vi "Problem_Track_Sorter-3.vi"(0 "[IN] Unsorted Tracks":dbl[][](array[numeric]), 1 "[IN] Dot matrix":i16[][](array[numeric]), 3 "error IN":errorcluster) -> (4 "Filtered Dot Stat Matrix":i16[][](array[numeric]), 5 "Sorted Tracks OUT":dbl[][](array[numeric]), 6 "Track ID OUT":u16[](array[numeric]), 7 "Start Pos OUT":i32[](array[numeric]), 8 "error OUT":errorcluster)   [LabVIEW 2013]
doc: "SubVI sorts the tracks and assigns them the same ID"
panel:
  out "ID-dot matrix OUT":u16[][](array[numeric])
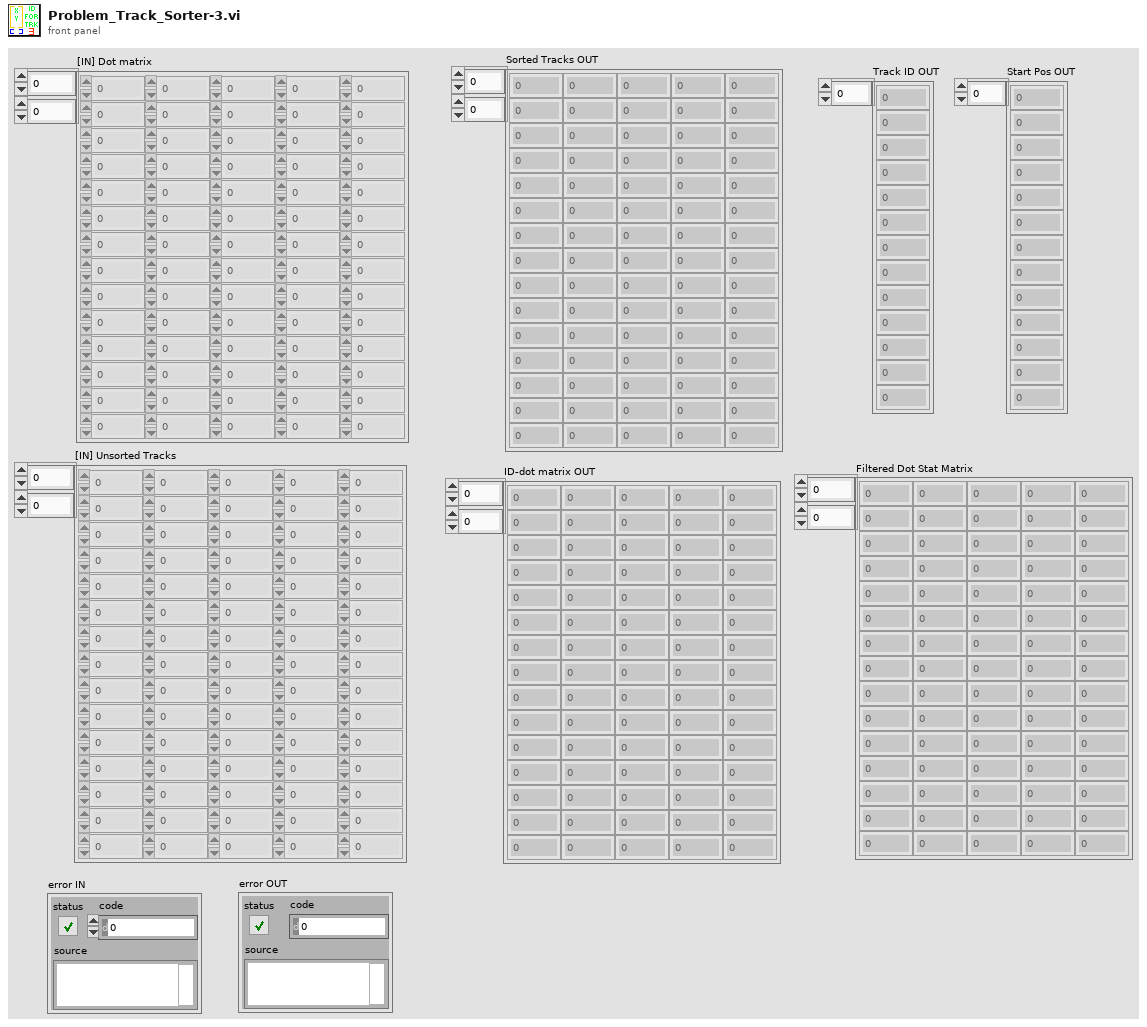
[diagram p1: front panel]
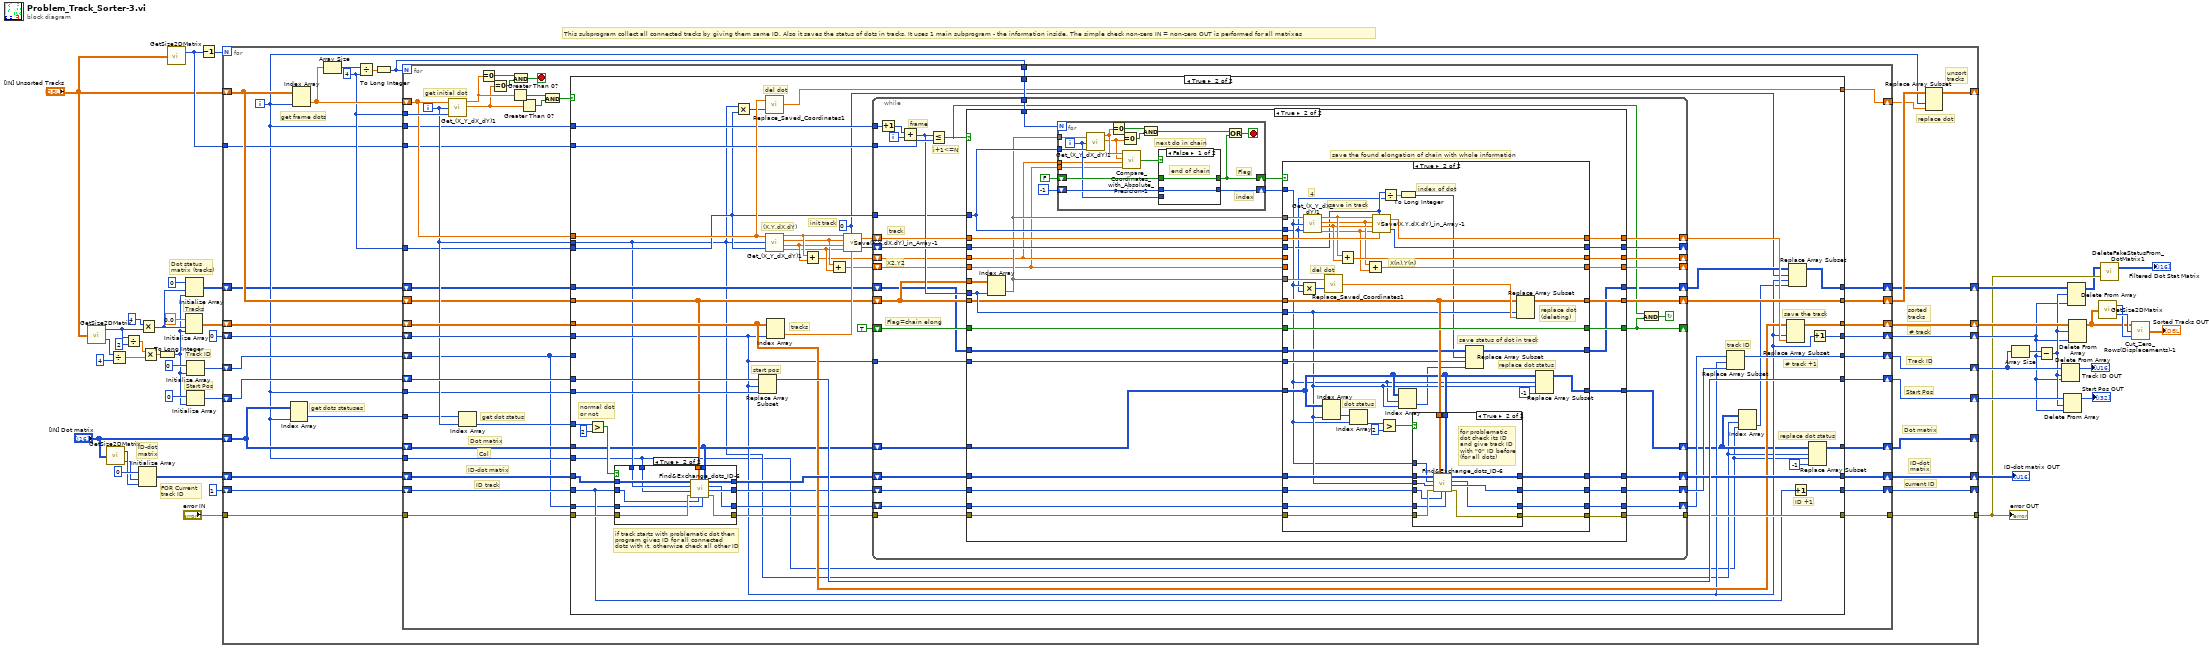
[diagram p0: block diagram]
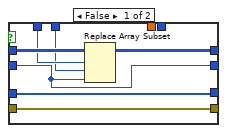
[diagram p3: hidden frame]
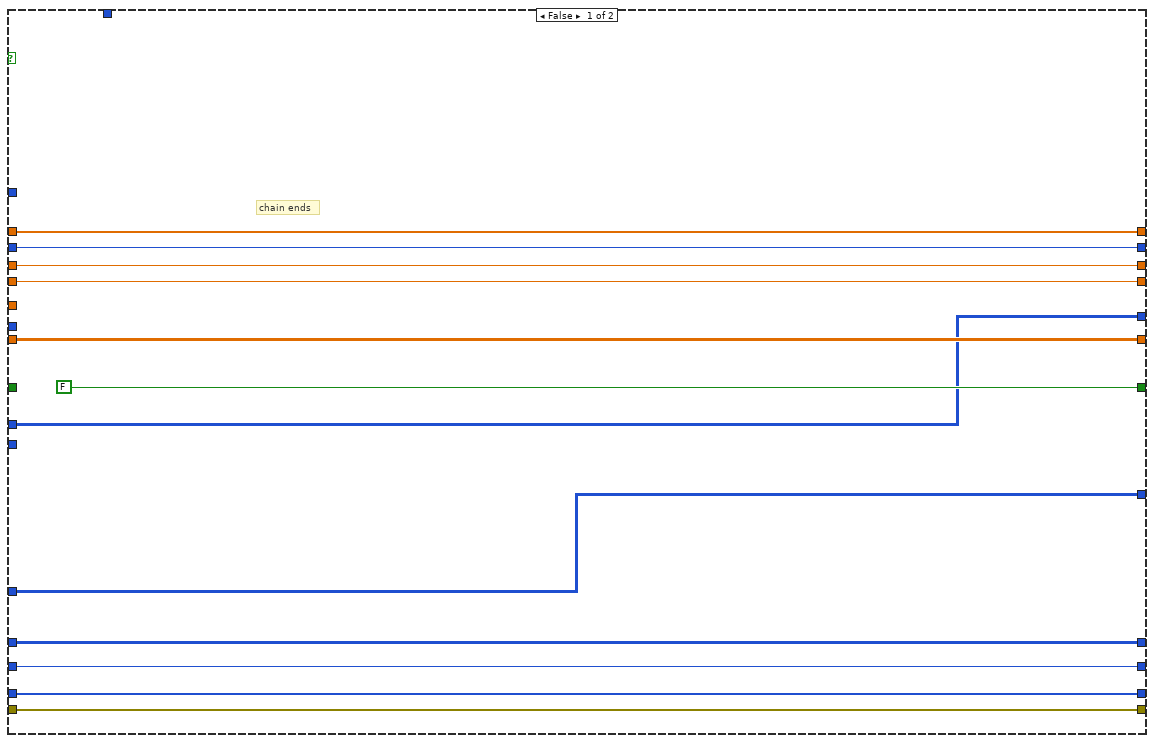
[diagram p4: hidden frame]
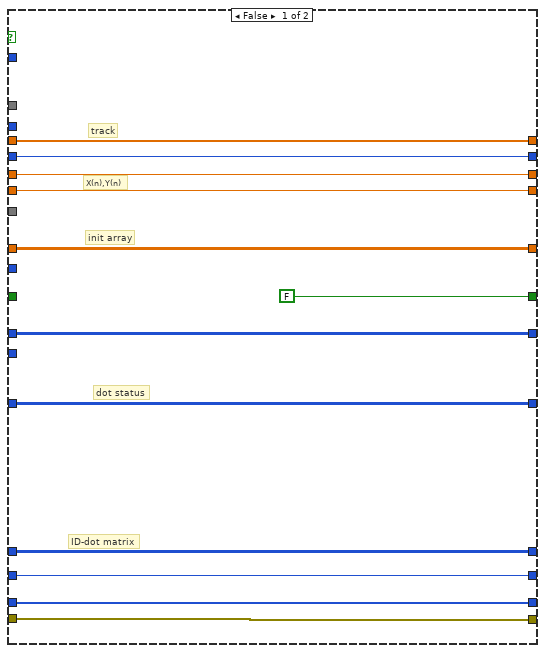
[diagram p5: hidden frame]
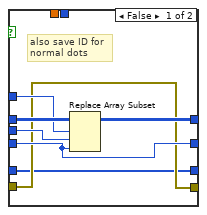
[diagram p6: hidden frame]
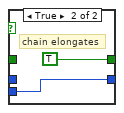
[diagram p7: hidden frame]
diagram:
  # "This subprogram collect all connected tracks by giving them same ID. Also it saves the status of dots in tracks. It uses 1 main subprogram - the information inside. The simple check non-zero IN = non-zero OUT is performed for all matrixes"
  # "Dot status\nmatrix (tracks)"
  # "FOR Current \ntrack ID"
  # "Start Pos"
  # "Track ID"
  # "Tracks"
  # "ID-dot\nmatrix"
  n1 = call "GetSize2DMatrix.vi"("Array IN (2D)"="[IN] Unsorted Tracks") -> ("# Cols"=w38:i32, "# Rows"=w40:i32)
  n2 = call "GetSize2DMatrix.vi"("Array IN (2D)"="[IN] Dot matrix") -> ("# Cols"=w44:i32, "# Rows"=w43:i32)
  n3 = Divide(x=w40, y=4) -> (x/y=w35:dbl)
  n4 = Divide(x=w38, y=2) -> (x/y=w36:dbl)
  n5 = Initialize Array(u16 0 ("element"), w43, w44) -> (w25:u16[][])
  n6 = Multiply(x=4, y=w38) -> (x*y=w10:i32)
  n7 = Multiply(x=w36, y=w35) -> (x*y=w34:dbl)
  n8 = To Long Integer(number=w34) -> (32bit integer=w9:i32)
  n9 = call "GetSize2DMatrix.vi"("Array IN (2D)"="[IN] Unsorted Tracks") -> ("# Cols"=w26:i32)  [unwired: 1 out]
  n10 = Initialize Array(0.0 ("element"), w10, w9) -> (w33:dbl[][])
  n11 = Initialize Array(i16 0, w10, w9) -> (w8:i16[][])
  n12 = Initialize Array(0 ("element"), w9) -> (w30:i32[])
  n13 = Initialize Array(u16 0 ("element"), w9) -> (w29:u16[])
  n14 = Decrement(x=w26) -> (x-1=w46:i32)
  n15 = for {
    N: w46 -> [_]
    shift-right: [w51] -> _
    shift-left: "[IN] Unsorted Tracks" -> [w65]
    shift-right: [w55] -> _
    shift-left: "[IN] Dot matrix" -> [w66]
    shift-right: [w58] -> w13
    shift-left: w33 -> [w71]
    shift-right: [w56] -> w19
    shift-left: w30 -> [w69]
    shift-right: [w57] -> w22
    shift-left: w29 -> [w70]
    shift-right: [w53] -> _
    shift-left: u16 1 -> [w72]
    shift-right: [w59] -> w5
    shift-left: 0 ("element") -> [w68]
    tunnel: w26 -> [w64]
    shift-right: [w54] -> w23
    shift-left: w25 -> [w62]
    tunnel: "error IN" -> [w61]
    tunnel: [w60] -> w4
    shift-right: [w47] -> w7
    shift-left: w8 -> [w48]
    i -> [w49]
    w67 = 4 ("y")
    # "replace dot"
    # "current ID"
    # "ID-dot\nmatrix"
    # "Dot matrix"
    # "Start Pos"
    # "Track ID"
    # "sorted \ntracks"
    # "unsort\ntracks"
    # "# track"
    # "get dots statuses"
    # "get frame dots"
    n16 = Index Array(array=w66, index (col)=w49) -> (element=w73:i16[])  [unwired: 1 in]
    n17 = Index Array(array=w65, index (col)=w49) -> (element=w74:dbl[])  [unwired: 1 in]
    n18 = Array Size(array=w74) -> (size(s)=w76:i32)
    n19 = Divide(x=w76, y=w67) -> (x/y=w75:dbl)
    n20 = To Long Integer(number=w75) -> (32bit integer=w63:i32)
    n21 = for {
      N: w63 -> [_]
      tunnel: w67 -> [w116]
      shift-right: [w84] -> w53
      shift-left: w72 -> [w92]
      shift-right: [w89] -> w58
      shift-left: w71 -> [w107]
      shift-right: [w87] -> w57
      shift-left: w70 -> [w79]
      shift-right: [w91] -> w56
      shift-left: w69 -> [w108]
      shift-right: [w88] -> w59
      shift-left: w68 -> [w106]
      tunnel: w67 -> [w101]
      shift-right: [w90] -> w52
      shift-left: w65 -> [w99]
      shift-right: [w86] -> w55
      shift-left: w66 -> [w80]
      tunnel: w49 -> [w98]
      tunnel: w49 -> [w97]
      tunnel: w64 -> [w96]
      tunnel: w63 -> [w95]
      tunnel: w49 -> [w94]
      shift-right: [w85] -> w54
      shift-left: w62 -> [w93]
      tunnel: w73 -> [w100]
      tunnel: w61 -> [w83]
      tunnel: [w82] -> w60
      shift-right: [w81] -> w50
      shift-left: w74 -> [w103]
      shift-right: [w77] -> w47
      shift-left: w48 -> [w78]
      i -> [w102]
      stop <- w113 stop-if-true
      # "Col"
      # "Dot matrix"
      # "ID-dot matrix"
      # "ID track"
      # "get dot status"
      # "get initial dot"
      n22 = call "Get_(X_Y_dX_dY)1.vi"("(X,Y,dX,dY)"=w103, "index"=w102, "multiplier"=w116) -> ("X"=w105:dbl, "Y"=w104:dbl)  [unwired: 2 out]
      n23 = Index Array(array=w100, index=w102) -> (element=w109:i16)
      n24 = Equal To 0?(x=w105) -> (x = 0?=w115:bool)
      n25 = Equal To 0?(x=w104) -> (x = 0?=w114:bool)
      n26 = Greater Than 0?(x=w105) -> (x > 0?=w112:bool)
      n27 = And(x=w115, y=w114) -> (x .and. y?=w113:bool)
      n28 = Greater Than 0?(x=w104) -> (x > 0?=w111:bool)
      n29 = And(x=w112, y=w111) -> (x .and. y?=w110:bool)
      n30 = case shown="True" w110 {
        tunnel: w109 -> [_ w182]
        tunnel: w79 -> [w123 _]
        tunnel: w108 -> [w127 w180]
        tunnel: w107 -> [w125 w151]
        tunnel: w106 -> [w124 w135]
        tunnel: w103 -> [w118 w179]
        tunnel: w102 -> [_ w131]
        tunnel: w101 -> [_ w145]
        tunnel: w80 -> [w122 w139]
        tunnel: w99 -> [w126 w144]
        tunnel: w98 -> [_ w178]
        tunnel: w97 -> [_ w177]
        tunnel: w96 -> [_ w176]
        tunnel: w95 -> [_ w175]
        tunnel: w94 -> [_ w130]
        tunnel: w93 -> [w121 w153]
        tunnel: w92 -> [w120 w143]
        tunnel: [w127 w172] -> w91
        tunnel: [w126 w174] -> w90
        tunnel: [w125 w169] -> w89
        tunnel: [w124 w168] -> w88
        tunnel: [w123 w173] -> w87
        tunnel: [w122 w138] -> w86
        tunnel: [w121 w171] -> w85
        tunnel: [w120 w170] -> w84
        tunnel: w83 -> [w119 w149]
        tunnel: [w119 w167] -> w82
        tunnel: [w118 w146] -> w81
        tunnel: w79 -> [_ w142]
        tunnel: w78 -> [w117 w137]
        tunnel: [w117 w128] -> w77
        frame False {
          # "fake dot! not counting"
        }
        frame True {
          w134 = 0
          # "if track starts with problematic dot then \nprogram gives ID for all connected\ndots with it, otherwise check all other ID"
          # "replace dot status"
          # "# track +1"
          # "ID +1"
          # "save the track"
          # "track ID"
          # "tracks"
          # "start pos"
          # "(X,Y,dX,dY)"
          # "init track"
          # "del dot"
          # "normal dot\nor not"
          n31 = Greater?(x=w182, y=i16 2) -> (0:w150:bool)
          n32 = case shown="True" w150 {
            tunnel: w143 -> [w185 w195]
            tunnel: w153 -> [w189 w199]
            tunnel: [w188 w190] -> w152
            tunnel: [w185 w192] -> w147
            tunnel: w149 -> [w184 w196]
            tunnel: [w184 w193] -> w148
            tunnel: w144 -> [_ w201]
            tunnel: w139 -> [_ w200]
            tunnel: w131 -> [w187 w198]
            tunnel: w130 -> [w186 w197]
            tunnel: [w183 w191] -> w141
            tunnel: w142 -> [w183 w194]
            frame False {
              n33 = Replace Array Subset(array=w189, new element=w185, index (row)=w187, index (col)=w186) -> (w188:u16[][])
            }
            frame True {
              n34 = call "Find&Exchange_dots_ID-6.vi"("Track ID Arr IN"=w194, "Dot matrix (stat)"=w200, "track ID IN"=w195, "(X,Y...) Tracks"=w201, "error IN"=w196, "frame (col)"=w197, "index of \ndot in frame"=w198, "ID-dot matrix"=w199) -> ("error OUT"=w193:errorcluster, "track ID OUT"=w192:u16, "Track ID Arr OUT"=w191:u16[], "ID-dot matrix OUT"=w190:u16[][])
            }
          }
          n35 = Multiply(x=w131, y=w145) -> (x*y=w165:i32)
          n36 = Replace Array Subset(array=w180, new element=w178, index=w135) -> (w172:i32[])
          n37 = call "Replace_Saved_Coordinates1.vi"("Index of staring point"=w165, "(X,Y,dX,dY) Frame IN"=w179) -> ("Replaced array"=w146:dbl[])
          n38 = call "Get_(X_Y_dX_dY)1.vi"("(X,Y,dX,dY)"=w179, "index"=w131, "multiplier"=w145) -> ("X"=w162:dbl, "Y"=w160:dbl, "dX"=w161:dbl, "dY"=w159:dbl)
          n39 = Index Array(array=w151, index (col)=w135) -> (element=w166:dbl[])  [unwired: 1 in]
          n40 = Add(x=w162, y=w161) -> (x+y=w158:dbl)
          n41 = Add(x=w160, y=w159) -> (x+y=w157:dbl)
          n42 = call "Save(X,Y,dX,dY)_in_Array-1.vi"("Array for Replacement IN"=w166, "Starting Position"=w134, "dY"=w159, "dX"=w161, "Y"=w160, "X"=w162) -> ("Finish Position"=w163:i32, "Array for Replacement OUT"=w164:dbl[])
          n43 = while {
            shift-right: [w221] -> w174
            shift-left: w144 -> [w222]
            shift-right: [w219] -> w154
            shift-left: w164 -> [w234]
            shift-right: [w218] -> _
            shift-left: w163 -> [w233]
            shift-right: [w212] -> w132
            shift-left: w139 -> [w217]
            tunnel: w177 -> [w231]
            tunnel: w176 -> [w235]
            shift-right: [w224] -> _
            shift-left: w158 -> [w228]
            shift-right: [w223] -> _
            shift-left: w157 -> [w227]
            tunnel: w175 -> [w226]
            tunnel: w145 -> [w225]
            shift-right: [w214] -> w171
            shift-left: w152 -> [w216]
            shift-right: [w210] -> _
            shift-left: TRUE -> [w220]
            shift-right: [w213] -> w155
            shift-left: w147 -> [w215]
            tunnel: w148 -> [w208]
            tunnel: [w207] -> w167
            shift-right: [w205] -> w140
            shift-left: w141 -> [w206]
            shift-right: [w202] -> w136
            shift-left: w137 -> [w204]
            tunnel: w135 -> [w203]
            i -> [w232]
            stop <- w211 continue-if-true
            # "i+1<=N"
            # "Flag=chain elong"
            # "frame"
            # "track"
            # "X2,Y2"
            n44 = Increment(x=w231) -> (x+1=w230:i32)
            n45 = Add(x=w230, y=w232) -> (x+y=w229:i32)
            n46 = Less Or Equal?(x=w229, y=w235) -> (x <= y?=w209:bool)
            n47 = case shown="True" w209 {
              tunnel: w222 -> [_ w272]
              tunnel: w234 -> [w247 w275]
              tunnel: w233 -> [w246 w274]
              tunnel: w229 -> [_ w271]
              tunnel: w228 -> [w245 w265]
              tunnel: w227 -> [w244 w264]
              tunnel: w226 -> [_ w281]
              tunnel: w225 -> [_ w276]
              tunnel: [w247 w269] -> w219
              tunnel: [w246 w268] -> w218
              tunnel: [w245 w267] -> w224
              tunnel: [w244 w266] -> w223
              tunnel: w222 -> [w243 w253]
              tunnel: [w243 w270] -> w221
              tunnel: w220 -> [_ w263]
              tunnel: [FALSE w262] -> w210
              tunnel: w217 -> [w240 w261]
              tunnel: w216 -> [w241 w260]
              tunnel: w215 -> [w239 w259]
              tunnel: [w241 w258] -> w214
              tunnel: [w239 w257] -> w213
              tunnel: [w240 w256] -> w212
              tunnel: w208 -> [w238 w255]
              tunnel: [w238 w254] -> w207
              tunnel: w206 -> [w237 w252]
              tunnel: [w237 w251] -> w205
              tunnel: w204 -> [w236 w250]
              tunnel: w203 -> [_ w249]
              tunnel: [w236 w248] -> w202
              frame False {
                # "chain ends"
              }
              frame True {
                # "save the found elongation of chain with whole information"
                n48 = Index Array(array=w272, index (col)=w271) -> (element=w273:dbl[])  [unwired: 1 in]
                n49 = for {
                  N: w281 -> [_]
                  tunnel: w273 -> [w369]
                  tunnel: w276 -> [w368]
                  tunnel: w265 -> [w356]
                  tunnel: w264 -> [w355]
                  shift-right: [w361] -> w278
                  shift-left: FALSE -> [w363]
                  shift-right: [w360] -> w277
                  shift-left: -1 -> [w362]
                  i -> [w359]
                  stop <- w364 stop-if-true
                  # "next do in chain"
                  # "index"
                  # "Flag"
                  n50 = call "Get_(X_Y_dX_dY)1.vi"("(X,Y,dX,dY)"=w369, "index"=w359, "multiplier"=w368) -> ("X"=w358:dbl, "Y"=w357:dbl)  [unwired: 2 out]
                  n51 = Equal To 0?(x=w358) -> (x = 0?=w367:bool)
                  n52 = Equal To 0?(x=w357) -> (x = 0?=w366:bool)
                  n53 = call "Compare_Coordinates_with_Absolute_Presicion-1.vi"("X 1"=w358, "Y 1"=w357, "X 2"=w356, "Y 2"=w355) -> ("[OUT] Same coordinates?"=w354:bool)  [unwired: 1 in]
                  n54 = And(x=w367, y=w366) -> (x .and. y?=w365:bool)
                  n55 = case shown="False" w354 {
                    tunnel: w363 -> [w371 _]
                    tunnel: w362 -> [w370 _]
                    tunnel: [w371 TRUE] -> w361
                    tunnel: [w370 w372] -> w360
                    tunnel: w359 -> [_ w372]
                    frame False {
                      # "end of chain"
                    }
                    frame True {
                      # "chain elongates"
                    }
                  }
                  n56 = Or(x=w365, y=w361) -> (x .or. y?=w364:bool)
                }
                n57 = case shown="True" w278 {
                  tunnel: w277 -> [_ w300]
                  tunnel: w273 -> [_ w334]
                  tunnel: w276 -> [_ w298]
                  tunnel: w275 -> [w293 w333]
                  tunnel: w274 -> [w292 w299]
                  tunnel: w273 -> [_ w331]
                  tunnel: w253 -> [w291 w307]
                  tunnel: w271 -> [_ w301]
                  tunnel: [w293 w329] -> w269
                  tunnel: [w292 w328] -> w268
                  tunnel: [w291 w311] -> w270
                  tunnel: [w290 w325] -> w267
                  tunnel: [w289 w322] -> w266
                  tunnel: w265 -> [w290 _]
                  tunnel: w264 -> [w289 _]
                  tunnel: [FALSE w321] -> w262
                  tunnel: w263 -> [_ w321]
                  tunnel: w261 -> [w287 w302]
                  tunnel: w260 -> [w285 w315]
                  tunnel: w259 -> [w286 w316]
                  tunnel: [w285 w314] -> w258
                  tunnel: [w287 w310] -> w256
                  tunnel: [w286 w312] -> w257
                  tunnel: w255 -> [w284 w309]
                  tunnel: [w284 w308] -> w254
                  tunnel: w252 -> [w283 w306]
                  tunnel: [w283 w305] -> w251
                  tunnel: w250 -> [w282 w304]
                  tunnel: w249 -> [_ w303]
                  tunnel: [w282 w294] -> w248
                  frame False {
                    # "ID-dot matrix"
                    # "dot status"
                    # "init array"
                    # "X(n),Y(n)"
                    # "track"
                  }
                  frame True {
                    # "index of dot"
                    # "4"
                    # "save status of dot in track"
                    # "replace dot status"
                    # "dot status"
                    # "X(n),Y(n)"
                    # "save in track"
                    # "replace dot\n(deleting)"
                    # "del dot"
                    n58 = Multiply(x=w300, y=w298) -> (x*y=w332:i32)
                    n59 = call "Get_(X_Y_dX_dY)1.vi"("(X,Y,dX,dY)"=w334, "index"=w300, "multiplier"=w298) -> ("X"=w327:dbl, "Y"=w324:dbl, "dX"=w326:dbl, "dY"=w323:dbl)
                    n60 = Index Array(array=w302, index (col)=w301) -> (element=w320:i16[])  [unwired: 1 in]
                    n61 = call "Replace_Saved_Coordinates1.vi"("Index of staring point"=w332, "(X,Y,dX,dY) Frame IN"=w331) -> ("Replaced array"=w330:dbl[])
                    n62 = Add(x=w327, y=w326) -> (x+y=w325:dbl)
                    n63 = Index Array(array=w320, index=w300) -> (element=w319:i16)
                    n64 = Add(x=w324, y=w323) -> (x+y=w322:dbl)
                    n65 = call "Save(X,Y,dX,dY)_in_Array-1.vi"("Array for Replacement IN"=w333, "Starting Position"=w299, "dY"=w323, "dX"=w326, "Y"=w324, "X"=w327) -> ("Finish Position"=w328:i32, "Array for Replacement OUT"=w329:dbl[])
                    n66 = Greater?(x=w319, y=i16 2) -> (0:w317:bool)
                    n67 = Divide(x=w299, y=w298) -> (x/y=w297:dbl)
                    n68 = Index Array(array=w302, index (row)=w300, index (col)=w301) -> (element=w295:i16)
                    n69 = To Long Integer(number=w297) -> (32bit integer=w296:i32)
                    n70 = case shown="True" w317 {
                      tunnel: w316 -> [w337 w346]
                      tunnel: w315 -> [w341 w350]
                      tunnel: w300 -> [w339 w349]
                      tunnel: w301 -> [w340 w347]
                      tunnel: [w338 w353] -> w314
                      tunnel: [w337 w343] -> w312
                      tunnel: w307 -> [_ w352]
                      tunnel: w302 -> [_ w351]
                      tunnel: w309 -> [w336 w348]
                      tunnel: [w336 w344] -> w308
                      tunnel: w306 -> [w335 w345]
                      tunnel: [w335 w342] -> w305
                      frame False {
                        # "also save ID for \nnormal dots"
                        n71 = Replace Array Subset(array=w341, new element=w337, index (row)=w339, index (col)=w340) -> (w338:u16[][])
                      }
                      frame True {
                        # "for problematic \ndot check its ID \nand give track ID \nwith \"0\" ID before \n(for all dots)"
                        n72 = call "Find&Exchange_dots_ID-6.vi"("Track ID Arr IN"=w345, "Dot matrix (stat)"=w351, "track ID IN"=w346, "(X,Y...) Tracks"=w352, "error IN"=w348, "frame (col)"=w347, "index of \ndot in frame"=w349, "ID-dot matrix"=w350) -> ("error OUT"=w344:errorcluster, "track ID OUT"=w343:u16, "Track ID Arr OUT"=w342:u16[], "ID-dot matrix OUT"=w353:u16[][])
                      }
                    }
                    n73 = Replace Array Subset(array=w304, new element=w295, index (row)=w296, index (col)=w303) -> (w294:i16[][])
                    n74 = Replace Array Subset(array=w307, new element=w330, index (col)=w301) -> (w311:dbl[][])  [unwired: 1 in]
                    n75 = Replace Array Subset(array=w302, new element=i16 -1 ("new element/subarray"), index (row)=w300, index (col)=w301) -> (w310:i16[][])
                  }
                }
              }
            }
            n76 = And(x=w209, y=w210) -> (x .and. y?=w211:bool)
          }
          n77 = Replace Array Subset(array=w140, new element=w155, index=w135) -> (w173:u16[])
          n78 = Index Array(array=w132, index (row)=w131, index (col)=w130) -> (element=w129:i16)
          n79 = Replace Array Subset(array=w151, new element=w154, index (col)=w135) -> (w169:dbl[][])  [unwired: 1 in]
          n80 = Replace Array Subset(array=w136, new element=w129, index (row)=w134, index (col)=w135) -> (w128:i16[][])
          n81 = Increment(x=w143) -> (x+1=w170:u16)
          n82 = Replace Array Subset(array=w132, new element=i16 -1 ("new element/subarray"), index (row)=w131, index (col)=w130) -> (w138:i16[][])
          n83 = Increment(x=w135) -> (x+1=w168:i32)
        }
      }
    }
    n84 = Replace Array Subset(array=w52, new element=w50, index (col)=w49) -> (w51:dbl[][])  [unwired: 1 in]
  }
  "error OUT" <- w4
  "ID-dot matrix OUT" <- w23
  n85 = Array Size(array=w22) -> (size(s)=w21:i32)
  n86 = Subtract(x=w21, y=w5) -> (x-y=w6:i32)
  n87 = Delete From Array(array=w22, length=w6, index=w5) -> (array with subset deleted=→"Track ID OUT":u16[])  [unwired: 1 out]
  n88 = Delete From Array(array=w19, length=w6, index=w5) -> (array with subset deleted=→"Start Pos OUT":i32[])  [unwired: 1 out]
  n89 = Delete From Array(array=w7, length=w6, index (col)=w5) -> (array with subset deleted=w3:i16[][])  [unwired: 1 in, 1 out]
  n90 = Delete From Array(array=w13, length=w6, index (col)=w5) -> (array with subset deleted=w15:dbl[][])  [unwired: 1 in, 1 out]
  n91 = call "GetSize2DMatrix.vi"("Array IN (2D)"=w15) -> ("# Cols"=w16:i32, "# Rows"=w17:i32)
  n92 = call "DeleteFakeStatusFrom_DotMatrix1.vi"("error IN"=w4, "Source Matrix"=w3) -> ("Filtered Dot Matrix"=→"Filtered Dot Stat Matrix":i16[][])  [unwired: 1 out]
  n93 = call "Cut_Zero_Rows(Displacements)-1.vi"("# Cols"=w16, "# Rows"=w17, "Array IN"=w15) -> ("Array OUT"=→"Sorted Tracks OUT":dbl[][])
